vi "GetParam.vi"(8 "error in (no error)":errorcluster caption="entrée d'erreur (pas d'erreur)", 11 "ShuffleSplit.lvclass":refnum<class "ShuffleSplit.lvclass">) -> (0 "error out":errorcluster caption="sortie d'erreur", 2 "ShuffleSplit":T1={"n_splits"=10, "test_size"="None", "train_size"="None", "random_state"=-1} {"random_state" min=-1}, 3 "ShuffleSplit.lvclass":refnum<class "ShuffleSplit.lvclass">)   [LabVIEW 2020, in "ShuffleSplit.lvclass"]
doc: "Get Parameters"
uses:
  ShuffleSplit.lvclass
  ShuffleSplit.lvclass/ShuffleSplit.ctl
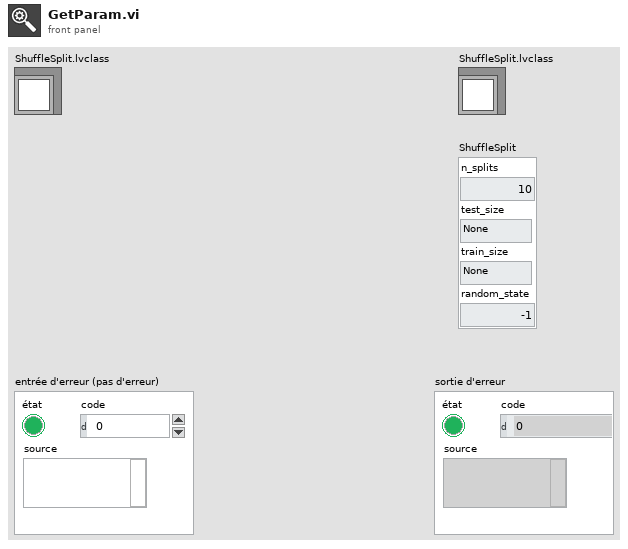
[diagram p1: front panel]
types:
  T1 = cluster{"n_splits":i32, "test_size":string, "train_size":string, "random_state":i32}
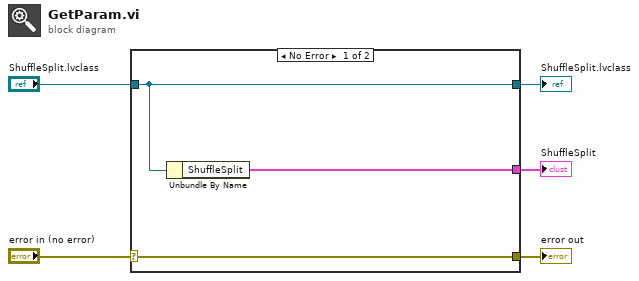
[diagram p0: block diagram]
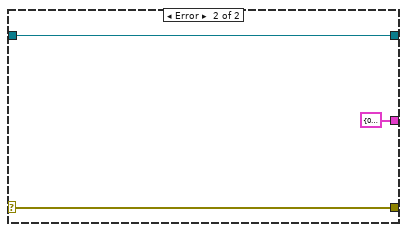
[diagram p2: hidden frame]
diagram:
  n1 = case shown="No Error" "error in (no error)" {
    selector: "error in (no error)" -> [w8 w10]
    tunnel: [w8 w10] -> w4
    tunnel: [w7 w11] -> w2
    tunnel: "ShuffleSplit.lvclass" -> [w7 w11]
    tunnel: [w6 T1 {"n_splits"=0, "test_size"="", "train_size"="", "random_state"=0} ("ShuffleSplit")] -> w1
    frame No Error {
      n2 = Unbundle By Name(w7) -> ("ShuffleSplit"=w6:T1)
    }
    frame Error {
    }
  }
  "error out" <- w4
  "ShuffleSplit.lvclass" <- w2
  "ShuffleSplit" <- w1
